vi "Destroy.vi"(0 "reference in":refnum<class "G#BaseTemplateG3.lvclass">, 5 "error in (no error)":errorcluster) -> (14 "reference out":refnum<class "G#BaseTemplateG3.lvclass">, 19 "error out":errorcluster)   [LabVIEW 2020, in "G#BaseTemplateG3.lvclass"]
doc: "Destructor."
uses:
  G#BaseTemplateG3.lvclass
  C:/ProjectGSharpDevelopment_2020-3/gsharp/VIPM/Files/vi.lib/addons/_AddQ/G#Object/G#Object.lvclass
  G#Object/G#Object.lvclass
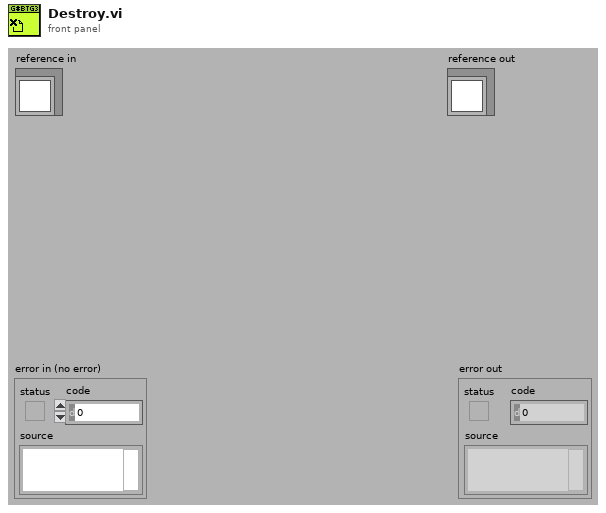
[diagram p1: front panel]
types:
  T1 = typedef "G#BaseTemplateG3.lvclass/ObjectAttributes.ctl" = cluster{"Numeric":dbl, "String":string, "Boolean":bool}
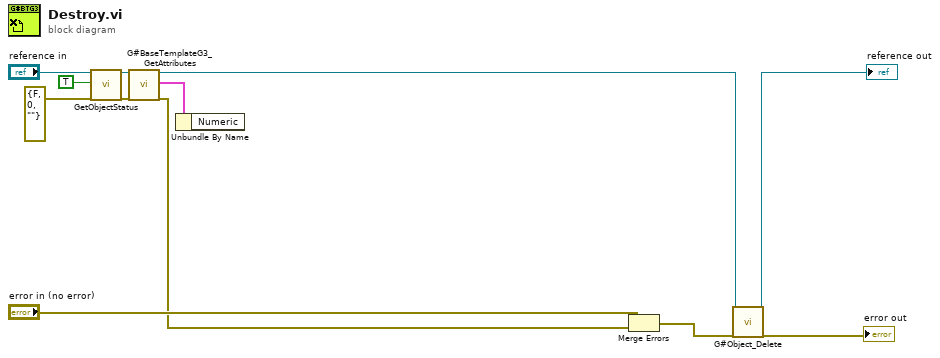
[diagram p0: block diagram]
diagram:
  n1 = call-dynamic "GetObjectStatus.vi"("reference in"="reference in", "simple info (F)"=TRUE ("simple info"), "error in (no error)"=errorcluster {"status"=FALSE, "code"=0, "source"=""}) -> ("reference out"=w6:refnum<class "G#BaseTemplateG3.lvclass">, "error out"=w4:errorcluster)  [unwired: 5 in, 10 out]
  n2 = call "G#BaseTemplateG3_GetAttributes.vi"("reference in"=w6, "error in (no error)"=w4) -> ("reference out"=w1:refnum<class "G#BaseTemplateG3.lvclass">, "attributes"=w8:T1, "error out"=w9:errorcluster)  [unwired: 14 in, 1 out]
  n3 = Unbundle By Name(w8) -> ()  [unwired: 1 out]
  n4 = Merge Errors("error in (no error)", w9) -> (w2:errorcluster)
  n5 = call "G#Object_Delete.vi"("reference in"=w1, "error in (no error)"=w2) -> ("reference out"=→"reference out":refnum<class "G#BaseTemplateG3.lvclass">, "error out"=→"error out":errorcluster)  [unwired: 16 in]
